vi "Initialize Control.vi"(8 "error in (no error)":errorcluster, 11 "QControl_Graph in":refnum<class "QControl_Graph.lvclass">) -> (0 "error out":errorcluster, 3 "QControl_Graph out":refnum<class "QControl_Graph.lvclass">)   [LabVIEW 2017, in "QControl_Graph.lvclass"]
doc: "The <b>Initialize VI</b> is a dynamic dispatch VI that must be overwritten in every QControl Class. It must <b>Call Parent Method</b> so that it recursively calls the initialize routine all of the way up the inheritance hierarchy. \n\nThe top most call is to the <b>Initialize Control VI</b> in Control.lvclass. This is the VI that starts the <b>Event Handler VI</b> if there was one overwritten in the QControl.\n<b> </b> <b> </b>\n©2016 Q Software Innovations, LLC (QSI)\nwritten by Quentin Alldredge\nproduced in LabVIEW 2015\n\nsupport@qsoftwareinnovations.com\nwww.qsoftwareinnovations.com\n\nAll rights reserved.\n\nRedistribution and use in source and binary forms, with or without modification, are permitted provided that the following conditions are met:\n\n * Redistributions of source code must retain the above copyright notice, this list of conditions and the following disclaimer.\n * Redistributions in binary form must reproduce the above copyright notice, this list of conditions and the following disclaimer in the documentation and/or other materials provided with the distribution.\n * Neither the name of Q Software Innovations, LLC. nor the names of its contributors may be used to endorse or promote products derived from this software without specific prior written permission.\n\nTHIS SOFTWARE IS PROVIDED BY THE COPYRIGHT HOLDERS AND CONTRIBUTORS \"AS IS\" AND ANY EXPRESS OR IMPLIED WARRANTIES, INCLUDING, BUT NOT LIMITED TO, THE IMPLIED WARRANTIES OF MERCHANTABILITY AND FITNESS FOR A PARTICULAR PURPOSE ARE DISCLAIMED. IN NO EVENT SHALL THE COPYRIGHT OWNER OR CONTRIBUTORS BE LIABLE FOR ANY DIRECT, INDIRECT, INCIDENTAL, SPECIAL, EXEMPLARY, OR CONSEQUENTIAL DAMAGES (INCLUDING, BUT NOT LIMITED TO, PROCUREMENT OF SUBSTITUTE GOODS OR SERVICES; LOSS OF USE, DATA, OR PROFITS; OR BUSINESS INTERRUPTION) HOWEVER CAUSED AND ON ANY THEORY OF LIABILITY, WHETHER IN CONTRACT, STRICT LIABILITY, OR TORT (INCLUDING NEGLIGENCE OR OTHERWISE) ARISING IN ANY WAY OUT OF THE USE OF THIS SOFTWARE, EVEN IF ADVISED OF THE POSSIBILITY OF SUCH DAMAGE."
uses:
  QControl_Graph.lvclass
  <vilib>/QSI/QControls/QControl Classes/XYGraph/XYGraph.lvclass
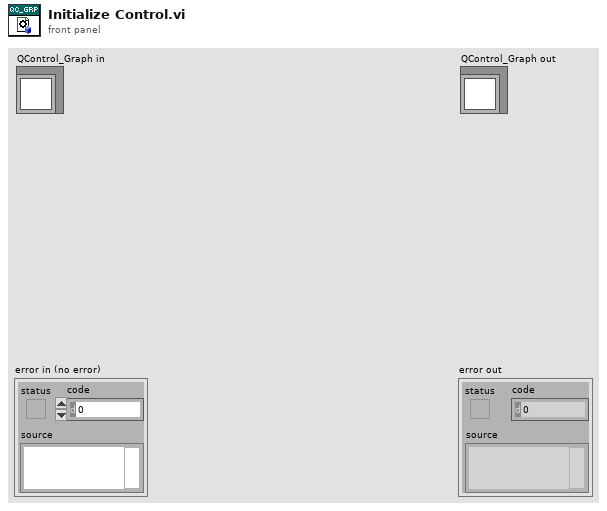
[diagram p1: front panel]
types:
  T1 = typedef "QControl_Graph.lvclass/Cursor Properties.ctl" = cluster{"font":T2, "size":i16, "time format (%H:%M:%S)":string, "Vertical Line?":bool, "Horizontal Line?":bool, "alignment(left, top)":T3, "TextFormat":string, "Timestamp":enum16{"at TOP", "at BOTTOM", "none"}}
  T2 = typedef "QControl_Graph.lvclass/Font.ctl" = cluster{"Font Name":string, "Size":i16, "Strikeout?":bool, "Italic?":bool, "Underline?":bool, "Outline?":bool, "Shadow":bool, "Bold?":bool}
  T3 = typedef "QControl_Graph.lvclass/Alignment.ctl" = cluster{"Horizontal":T4, "Vertical":T5}
  T4 = typedef "QControl_Graph.lvclass/Alignment.Horizontal.ctl" = enum16{"left", "center", "right"}
  T5 = typedef "QControl_Graph.lvclass/Alignment.Vertical.ctl" = enum16{"top", "center", "bottom"}
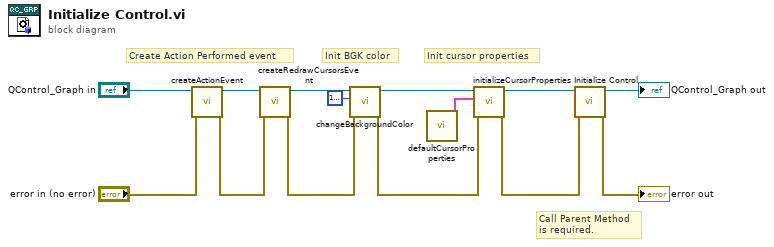
[diagram p0: block diagram]
diagram:
  # "Init cursor properties"
  # "Init BGK color"
  # "Create Action Performed event"
  # "Call Parent Method\nis required."
  n1 = call-dynamic "createActionEvent.vi"("error in (no error)"="error in (no error)", "QControl_Graph in"="QControl_Graph in") -> ("error out"=w2:errorcluster, "QControl_Graph out"=w4:refnum<class "QControl_Graph.lvclass">)  [unwired: 8 in]
  n2 = call-dynamic "createRedrawCursorsEvent.vi"("error in (no error)"=w2, "QControl_Graph in"=w4) -> ("error out"=w1:errorcluster, "QControl_Graph out"=w3:refnum<class "QControl_Graph.lvclass">)  [unwired: 8 in]
  n3 = call-dynamic "changeBackgroundColor.vi"("error in (no error)"=w1, "Color (transparent)"=u32 16777226, "QControl_Graph in"=w3) -> ("error out"=w7:errorcluster, "QControl_Graph out"=w9:refnum<class "QControl_Graph.lvclass">)  [unwired: 7 in]
  n4 = call "defaultCursorProperties.vi"() -> ("Default Cursor Properties"=w5:T1)  [unwired: 11 in]
  n5 = call-dynamic "initializeCursorProperties.vi"("error in (no error)"=w7, "Cursor Properties"=w5, "QControl_Graph in"=w9) -> ("error out"=w6:errorcluster, "QControl_Graph out"=w8:refnum<class "QControl_Graph.lvclass">)  [unwired: 7 in]
  n6 = call-parent "Initialize Control.vi"("error in (no error)"=w6, "Control in"=w8) -> ("error out"=→"error out":errorcluster, "Control out"=→"QControl_Graph out":refnum<class "QControl_Graph.lvclass">)  [unwired: 8 in]
